vi "Drive.vi"(10 "Drive Loop State":T1) -> ()   [LabVIEW 2018]
uses:
  DriveLoopEnum.ctl
  driveShiftEnum.ctl
  <vilib>/Rock Robotics/WPI/ThirdParty/Phoenix-LabVIEW/Motor Controller/Controls/CTRE_Phoenix_MotorControl_ControlMode.ctl
  <vilib>/Rock Robotics/WPI/Utilities/WPI_GetSetVariantRefNum.vi
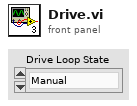
[diagram p1: front panel]
types:
  T1 = typedef "DriveLoopEnum.ctl" = enum16{"Manual", "Motion Magic"}
  T2 = typedef "WPI_JoystickDevRef.ctl" = cluster{"Device":T3}
  T3 = typedef "WPI_JoystickDeviceEnum.ctl" = enum16{"USB 0", "USB 1", "USB 2", "USB 3", "USB 4", "USB 5"}
  T4 = typedef "WPI_MotorControlDeviceRef.ctl" = cluster{"DeviceStatus":errorcluster, "Type":T5, "PWM":cluster{"PWM Channel":T6, "DeadBand":T7}, "CAN":cluster{"Device Number":u8, "SetOutput VI Ref":variant, "GetOutput VI Ref":variant, "Enable VI Ref":variant, "Disable VI Ref":variant, "Data":variant}, "Invert":bool, "DIO PWM":cluster{"PWM \"Enable\" Channel":T6, "DIOChannel":T8, "PWM Rate":dbl}}
  T5 = typedef "WPI_MotorControlType.ctl" = enum16{"PWM", "CAN", "DIO PWM"}
  T6 = typedef "FPGA_DIOPWMChannel.ctl" = enum8{"PWM 0", "PWM 1", "PWM 2", "PWM 3", "PWM 4", "PWM 5", "PWM 6", "PWM 7", "PWM 8", "PWM 9", "PWM MXP 0", "PWM MXP 1", "PWM MXP 2", "PWM MXP 3", "PWM MXP 4", "PWM MXP 5", "PWM MXP 6", "PWM MXP 7", "PWM MXP 8", "PWM MXP 9", "Invalid"}
  T7 = typedef "WPI_PWMDeadband.ctl" = cluster{"Name":string, "maxPositivePwm":i32, "minPositivePwm":i32, "centerPwm":i32, "maxNegativePwm":i32, "minNegativePwm":i32, "angularRange":u16}
  T8 = typedef "FPGA_DIOChannel.ctl" = enum8{"DIO 0", "DIO 1", "DIO 2", "DIO 3", "DIO 4", "DIO 5", "DIO 6", "DIO 7", "DIO 8", "DIO 9", "DIO MXP 0", "DIO MXP 1", "DIO MXP 2", "DIO MXP 3", "DIO MXP 4", "DIO MXP 5", "DIO MXP 6", "DIO MXP 7", "DIO MXP 8", "DIO MXP 9", "DIO MXP 10", "DIO MXP 11", "DIO MXP 12", "DIO MXP 13", "DIO MXP 14", "DIO MXP 15", "SPI Port CS1", "SPI Port CS2", "SPI Port CS3", "SPI Port MISO", "SPI Port MOSI", "Invalid"}
  T9 = typedef "driveShiftEnum.ctl" = enum16{"Low", "High"}
  T10 = typedef "CTRE_Phoenix_MotorControl_ControlMode.ctl" = u16
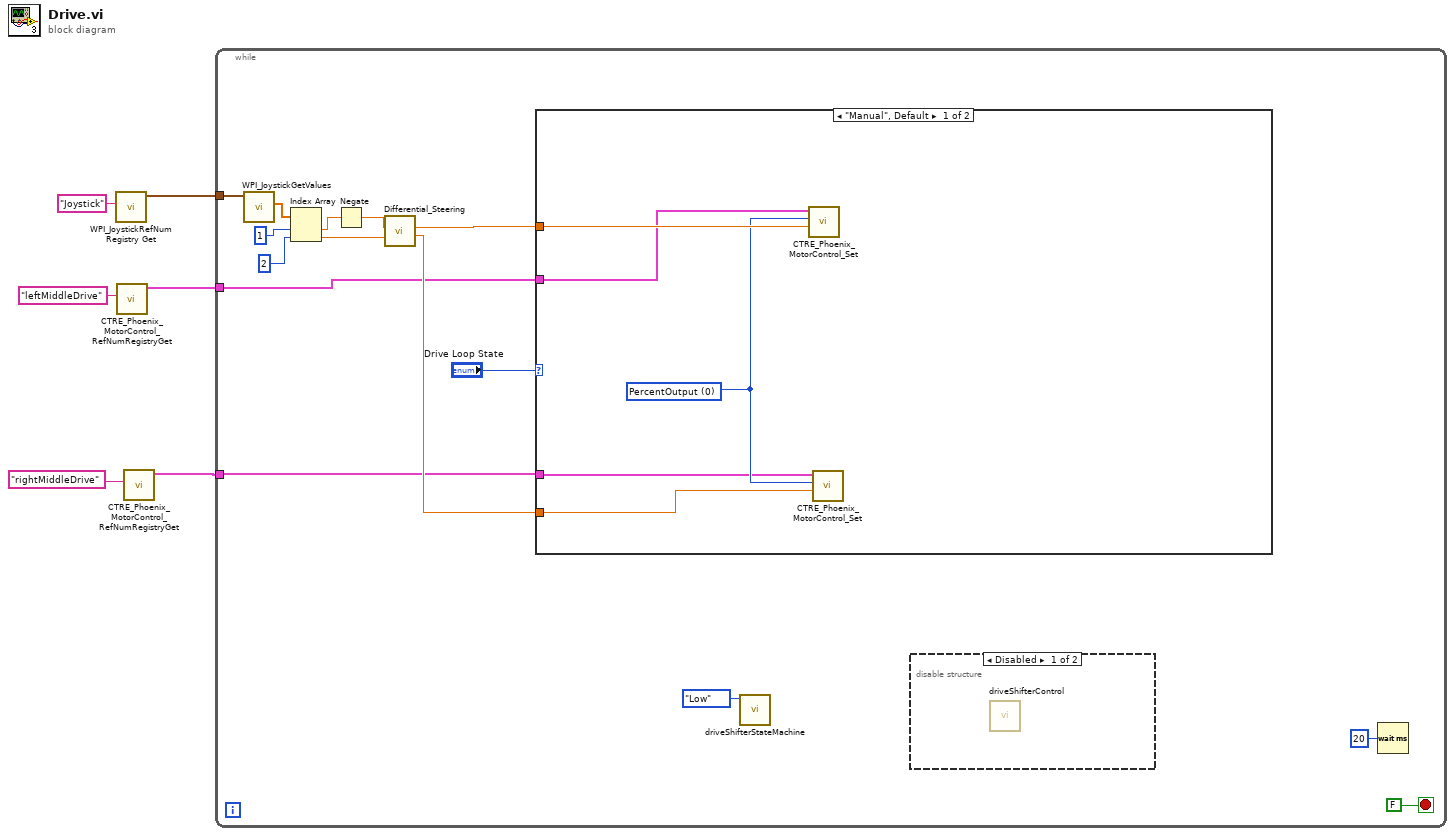
[diagram p0: block diagram]
diagram:
  n1 = call <vilib>:"WPI_JoystickRefNum Registry Get.vi"("refnum name"="Joystick") -> ("JoystickDevRef"=w5:T2)  [unwired: 9 in, 1 out]
  n2 = call <vilib>:"CTRE_Phoenix_MotorControl_RefNumRegistryGet.vi"("refnum name"="leftMiddleDrive") -> ("PhoenixMotorControlDevRef"=w2:T4)  [unwired: 9 in, 1 out]
  n3 = call <vilib>:"CTRE_Phoenix_MotorControl_RefNumRegistryGet.vi"("refnum name"="rightMiddleDrive") -> ("PhoenixMotorControlDevRef"=w1:T4)  [unwired: 9 in, 1 out]
  n4 = while {
    tunnel: w5 -> [w17]
    tunnel: w2 -> [w11]
    tunnel: w1 -> [w10]
    stop <- FALSE stop-if-true
    n5 = call <vilib>:"WPI_JoystickGetValues.vi"("JoystickDevRef"=w17) -> ("Axes"=w15:dbl[])  [unwired: 6 in, 4 out]
    n6 = Index Array(array=w15, index #1=1 ("index"), index #2=2 ("index")) -> (element #1=w16:dbl, element #2=w14:dbl)
    n7 = Negate(x=w16) -> (-x=w9:dbl)
    n8 = call <userlib>:"Differential_Steering.vi"("Steer"=w14, "Base"=w9) -> ("Right"=w13:dbl, "Left"=w12:dbl)  [unwired: 4 in]
    n9 = case shown="\"Manual\", Default" "Drive Loop State" {
      tunnel: w13 -> [w26 _]
      tunnel: w12 -> [w25 _]
      tunnel: w11 -> [w23 _]
      tunnel: w10 -> [w22 _]
      frame "Manual", Default {
        w24 = T10 0 items=["PercentOutput"=0, "Position"=1, "Velocity"=2, "Current"=3, "Follower"=5, "MotionProfile"=6, "MotionMagic"=7, "MotionProfileArc"=10, "Disabled"=15] ("Control Mode")
        n10 = call <vilib>:"CTRE_Phoenix_MotorControl_Set.vi"("Output"=w25, "Control Mode"=w24, "PhoenixMotorControlDevRef"=w23) -> ()  [unwired: 7 in, 2 out]
        n11 = call <vilib>:"CTRE_Phoenix_MotorControl_Set.vi"("Output"=w26, "Control Mode"=w24, "PhoenixMotorControlDevRef"=w22) -> ()  [unwired: 7 in, 2 out]
      }
      frame "Motion Magic" {
      }
    }
    n12 = call "driveShifterStateMachine.vi"("Drive Shift State"=driveShiftEnum."Low") -> ()  [unwired: 11 in]
    n13 = disable-structure shown="Disabled" {
      frame Disabled {
        n14 = call "driveShifterControl.vi"() -> ()  [unwired: 12 in]
      }
      frame Enabled {
      }
    }
    n15 = Wait (ms)(milliseconds to wait=u32 20) -> ()  [unwired: 1 out]
  }
